vi "Scan_Hopping multiple CV at Surface.vi"() -> ()   [LabVIEW 2023]
uses:
  Sub_Vi/TypeDefs/Settings.ctl
  Sub_Vi/TypeDefs/ChangeOnFly.ctl
  Sub_Vi/TypeDefs/Display.ctl
  Sub_Vi/TypeDefsControls/Feedback Type.ctl
  Sub_Vi/TypeDefsControls/Time.ctl
  Settings.vi
panel:
  in  "No. of Cycles":i32=1 min=0
  in  "Feedback Type":T1
  in  "ABSOLUTE Distance To Retrack \nat line end /um":dbl=1.0
  out "Estimated Time (mins)":dbl
  in  "Retract After Scan":bool=TRUE
  in  "Post CV Time / s":dbl
  in  "Post Clean _Pre CV Time / s":dbl
  in  "Clean Time / s":dbl
  in  "V 4":dbl
  in  "V 3":dbl
  in  "Input Cluster":T2={"Scan Rate (um/s)"=15.0, "X Start"=15.0, "X End"=15.0, "Y Start"=15.0, "Y End"=15.0, " Z Start"=15.0, "HoppingDistance"=1.0, "V"=15.0, "Z End"=15.0, "Approach Rate Hopping (um/s)"=15.0, "Retrack Rate (um/s)"=15.0, "V 2"=15.0, "Approach Rate (um/s)"=15.0, "V 3"=15.0, "CV Rate / V/s"=15.0, "V 4"=15.0, "V 1"=15.0, "HoldTime1/s"=15.0, "Hold time 2 / s"=15.0, "Hold time 3/ s"=15.0, "No. of Cycles"=15}
  in  "Display Cluster":T3
  in  "ChangeonFly":T4
  in  "SettingsCluster":T5={"Sample Rate (us)"=1, "Samples Per Data Point (int, power of 2)"=1000, "DistanceToBulk (um)"=1000.0, "HoldTimeScaler"=0, "SaveData"=TRUE, "DistanceToBulk (um) 2"=-1.0, "DistanceToBulk (um) 3"=-1.0}
  in  "Greater Than":bool=TRUE
  out "XY Graph 3":cluster{"Y":dbl[], "Y":dbl[]}[](graph)
  out "XY Graph 2":cluster{"Y":dbl[], "Y":dbl[]}[](graph)
  in  "CV Rate / V/s":dbl=0.1 min=0.0
  in  "V2":dbl=1.0
  in  "V1":dbl
  in  "Approach Rate Hopping (um/s)":dbl=1.0
  in  "Retrack Rate (um/s)":dbl=1.0
  in  "HoppingDistance":dbl=1.0
  in  "Z End":dbl=38.0
  in  "ABSOLUTE Distance To Retrack / um":dbl=1.0
  in  "Upper dZ limit":i32=8
  in  "Feedback Threshold\nAbsolute value":dbl=1e-13
  in  "P":fxp<+/-,32,1> format="%.32g"
  in  "X Center":dbl=150.0 min=0.0 max=300.0
  in  "Y Center":dbl=150.0 min=0.0 max=300.0
  in  "Y Width":dbl=10.0
  in  "X Width":dbl=10.0
  in  "Scan Rate (um/s)":dbl=1.0
  in  "V":dbl=1.0
  in  "Approach Rate (um/s)":dbl=1.0
  in  "Z Start height":dbl
  in  "Start scan Button":bool
  in  "Stop":bool
  in  "Pause":bool
  in  "Start Scanning Button":bool
  out "Y end":dbl
  out "X end":dbl
  out "X start":dbl
  out "Y start":dbl
  in  "Tab Control 4":T6(tab)
  out "Topography":dbl[][](graph)
  out "Current 1":dbl[][](graph)
  out "Current 2":dbl[][](graph)
  out "Current 3":dbl[][](graph)
  out "Waveform Graph 2":dbl[](graph)
  out "Waveform Graph":dbl[](graph)
  out "XY Graph":cluster{"Y":dbl[], "Y":dbl[]}[](graph)
  out "Waveform Graph 4":dbl[](graph)
  out "Waveform Graph 3":dbl[](graph)
  # "Feedback  Settings"
  # "Approach  Settings"
  # "Scan  Settings"
  # "CV rate must not be zero"
  # "Define Scan area \nAbout centre"
  # "No. of Cycles"
  # "V3"
  # "V1"
  # "Clean Time / s"
  # "V"
  # "V"
  # "Jump to V"
  # "Approach"
  # "CV Rate"
  # "CV Rate"
  # "Post CV Time"
  # "Retract"
  # "V2"
  # "Post Clean Pre CV Time"
  # "V2"
  # "V4"
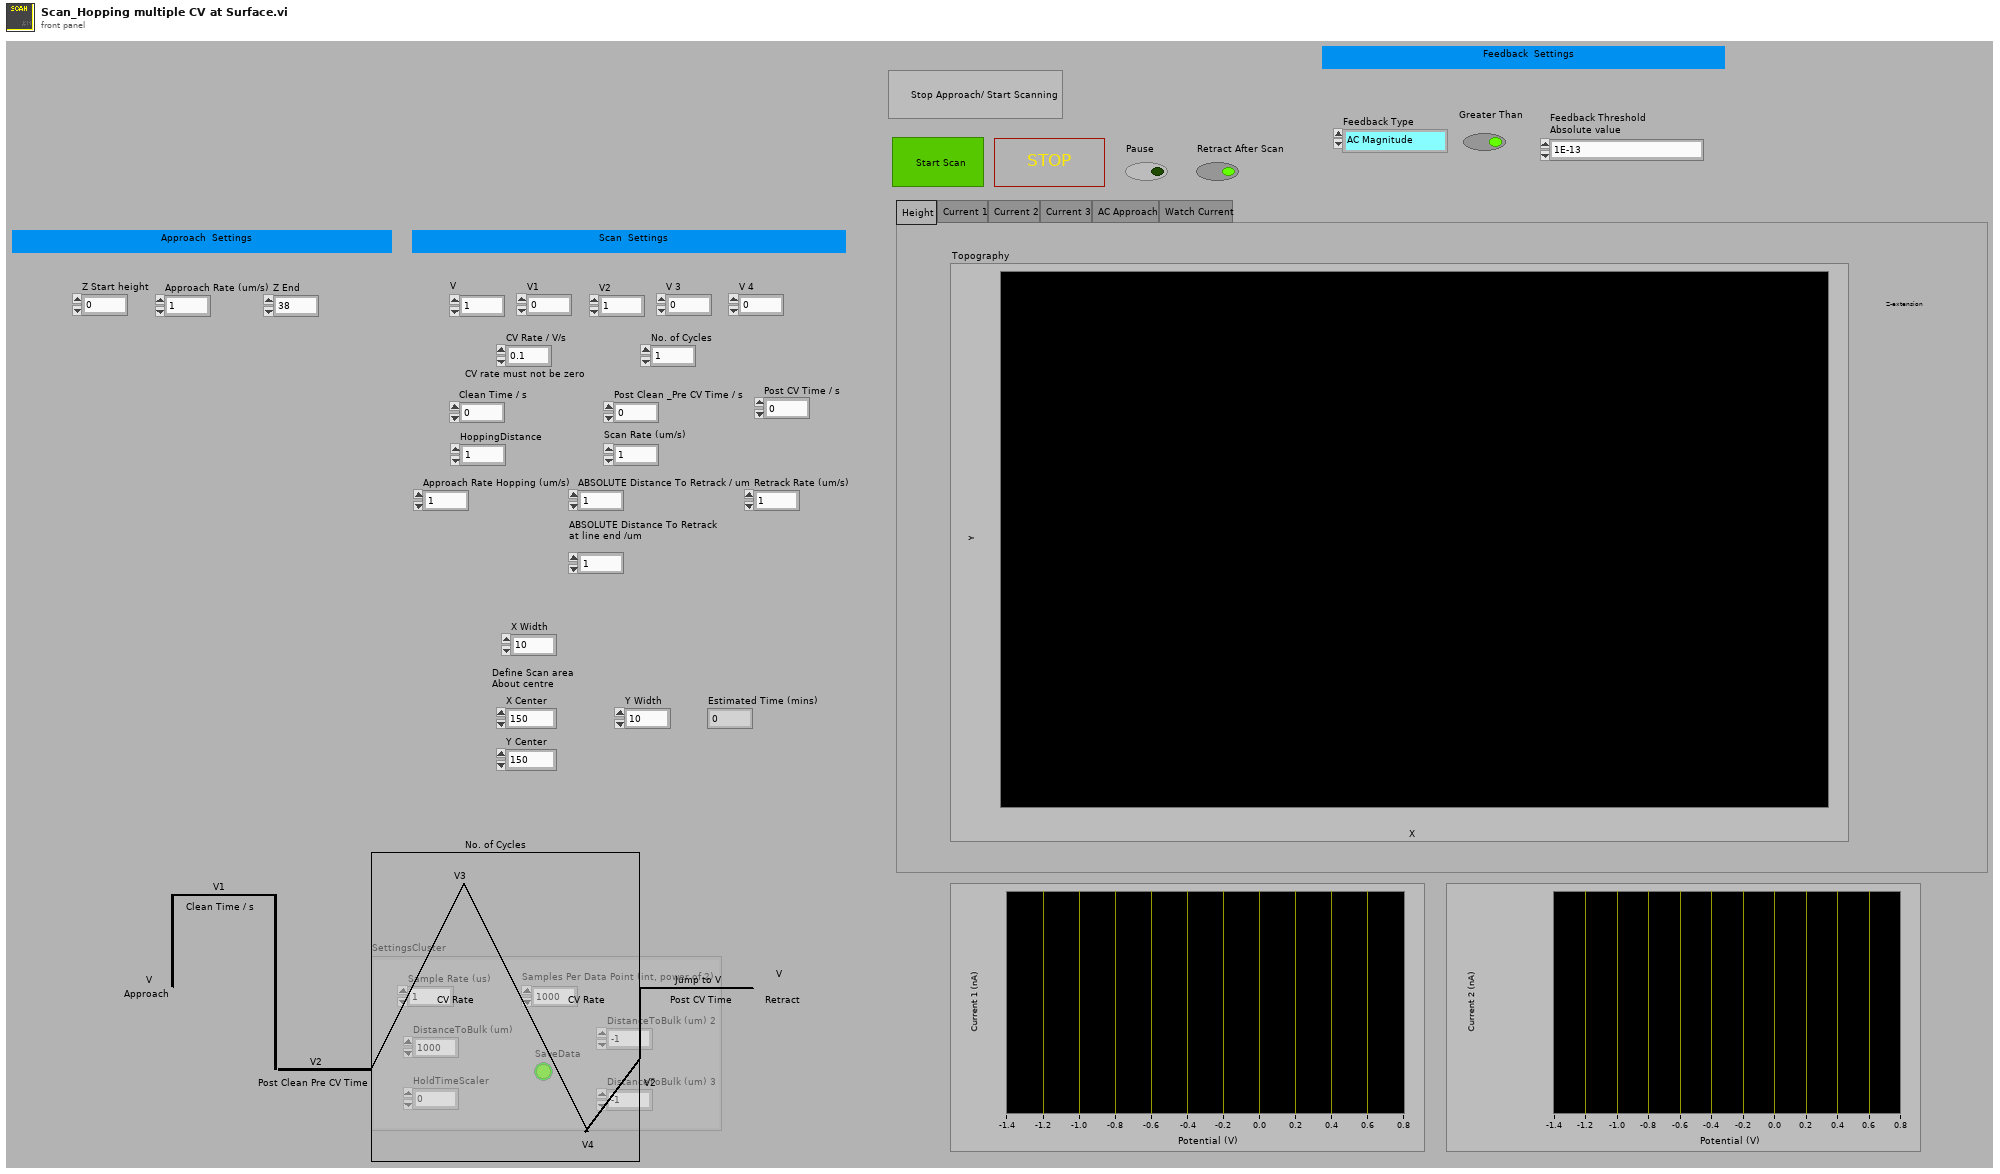
[diagram p1: front panel]
types:
  T1 = typedef "Feedback Type.ctl" = enum16{"AC Magnitude", "Current 1", "Current 2", "Phase"}
  T2 = cluster{"Scan Rate (um/s)":dbl, "X Start":dbl, "X End":dbl, "Y Start":dbl, "Y End":dbl, " Z Start":dbl, "HoppingDistance":dbl, "V":dbl, "Z End":dbl, "Approach Rate Hopping (um/s)":dbl, "Retrack Rate (um/s)":dbl, "V 2":dbl, "Approach Rate (um/s)":dbl, "V 3":dbl, "CV Rate / V/s":dbl, "V 4":dbl, "V 1":dbl, "HoldTime1/s":dbl, "Hold time 2 / s":dbl, "Hold time 3/ s":dbl, "No. of Cycles":i32}
  T3 = typedef "Display.ctl" = cluster{"X":refnum<vi>, "Y":refnum<vi>, "Z":refnum<vi>, "Amp":refnum<vi>, "Phase":refnum<vi>, "t vs Z":refnum<vi>, "t vs C1":refnum<vi>, "t vs C2":refnum<vi>, "t vs C3":refnum<vi>, "t vs Amp":refnum<vi>, "t vs Phase":refnum<vi>, "t vs X":refnum<vi>, "t vs Y":refnum<vi>, "Z vs C1":refnum<vi>, "Z vs C2":refnum<vi>, "Z vs C3":refnum<vi>, "V vs C1":refnum<vi>, "V vs C2":refnum<vi>, "V vs C3":refnum<vi>, "X/Y/Z F":refnum<vi>, "X/Y/Z R":refnum<vi>, "X/Y/C1 F":refnum<vi>, "X/Y/C1 R":refnum<vi>, "X/Y/C2 F":refnum<vi>, "X/Y/C2 R":refnum<vi>, "X/Y/C3 F":refnum<vi>, "X/Y/C3 R":refnum<vi>, "NumberOfLines":u16, "um Per Pixel":dbl, "um Per Line":dbl, "X Center":dbl, "Hop X/Y/Z":refnum<vi>, "Hop X/Y/C1":refnum<vi>, "Hop X/Y/C2":refnum<vi>, "Hop X/Y/C3":refnum<vi>, "X Width":dbl, "Y Width":dbl, "Hopping Distance":dbl, "V2 vs C1":refnum<vi>, "V vs Phase":refnum<vi>, "Y Center":dbl, "Number of Pixels":dbl, "V2 vs C2":refnum<vi>, "V2 vs C3":refnum<vi>, "V vs y":refnum<vi>, "V2 vs y":refnum<vi>, "Z vs Amp":refnum<vi>, "Z vs Phase":refnum<vi>}
  T4 = typedef "ChangeOnFly.ctl" = cluster{"Stop (boolean)":refnum<vi>, "Pause (boolean)":refnum<vi>, "EndCurrentLine (boolean)":refnum<vi>, "max movement per update step (Interger, nm)":refnum<vi>, "P (float, arb)":refnum<vi>, "Feedback set point (double, Amps)":refnum<vi>, "Voltage (double, V)":refnum<vi>, "Feedback set point 2 (double, Amps)":refnum<vi>, "Stop on Greater Than 2? (boolean)":refnum<vi>, "Stop on Greater Than? (boolean)":refnum<vi>, "Voltage 2 (double, V)":refnum<vi>, "Feedback Type (enum)":refnum<vi>, "Feedback Type 2 (enum)":refnum<vi>}
  T5 = typedef "Settings.ctl" = cluster{"Sample Rate (us)":u32, "Samples Per Data Point (int, power of 2)":i16, "DistanceToBulk (um)":dbl, "HoldTimeScaler":u64, "SaveData":bool, "DistanceToBulk (um) 2":dbl, "DistanceToBulk (um) 3":dbl}
  T6 = enum32{"Height", "Current 1", "Current 2", "Current 3", "AC Approach", "Watch Current"}
  T7 = typedef "Time.ctl" = dbl
  T8 = typedef "WayPointCluster.ctl" = cluster{"X (um)":dbl[], "Y (um)":dbl[], "Z (um)":dbl[], "V (V)":dbl[], "X Velocity (um s-1)":dbl[], "Y Velocity (um s-1)":dbl[], "Z Velocity (um s-1)":dbl[], "V Velocity (V s-1)":dbl[], "FeedBack Type (enum)":u16[], "Move X (boolean)":bool[], "Move Y (boolean)":bool[], "Move Z (boolean)":bool[], "Move V (boolean)":bool[], "Jump V (boolean)":bool[], "Hold (boolean)":bool[], "Hold Time":u32[], "V2 (V)":dbl[], "Move V2":bool[], "V2 Velocity (V s-1)":dbl[], "Jump V2 (boolean)":bool[], "Update z Position delta (ms)":i16[], "Hold Feedback1":bool[], "Move Z PicoMotor":bool[], " Z PicoMotor Direction":bool[], "DIO0":bool[]}
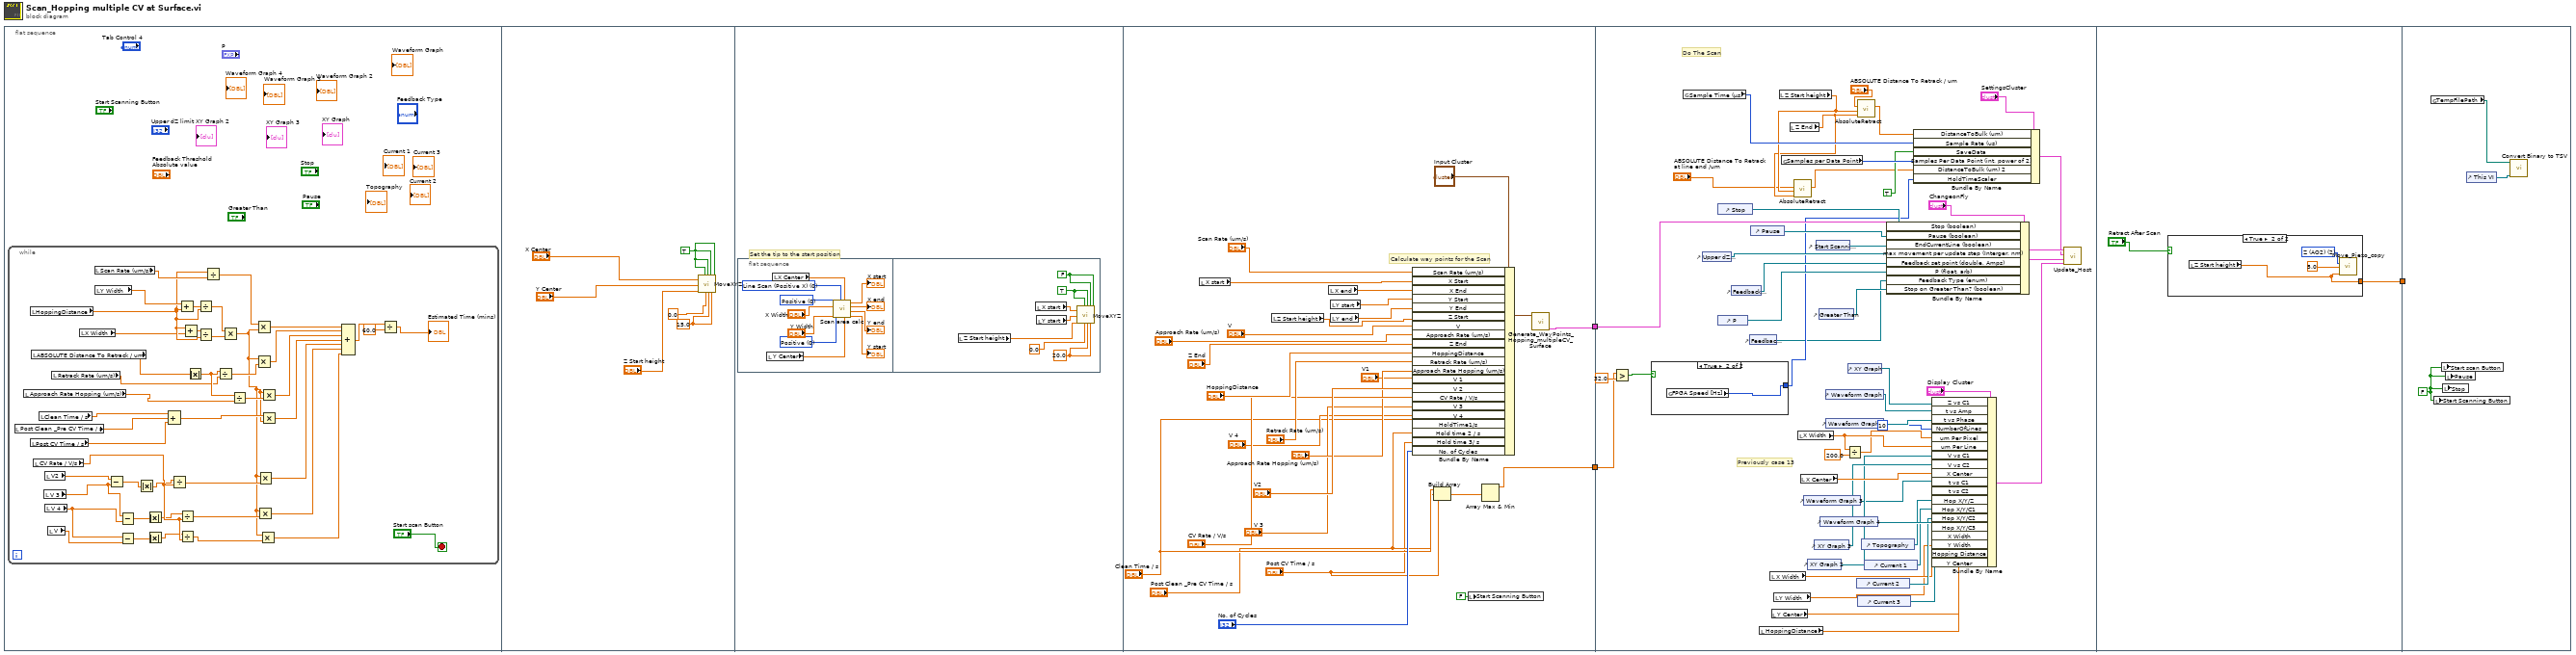
[diagram p0: block diagram]
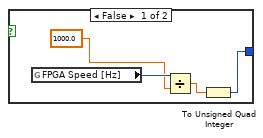
[diagram p2: hidden frame]
diagram:
  n1 = flat-sequence {
    tunnel: [w86] -> w3
    tunnel: [w73] -> w1
    tunnel: w3 -> [w112]
    tunnel: w1 -> [w101]
    tunnel: [w154] -> w2
    tunnel: w2 -> [_]
    frame #0 {
      n2 = while {
        stop <- "Start scan Button" stop-if-true
        n3 = local read "Post Clean _Pre CV Time / s"() -> (w17:dbl)
        n4 = local read "Approach Rate Hopping (um/s)"() -> (w20:dbl)
        n5 = local read "HoppingDistance"() -> (w23:dbl)
        n6 = local read "Post CV Time / s"() -> (w16:dbl)
        n7 = local read "ABSOLUTE Distance To Retrack / um"() -> (w21:dbl)
        n8 = local read "CV Rate / V/s"() -> (w7:dbl)
        n9 = local read "Clean Time / s"() -> (w18:dbl)
        n10 = local read "V 3"() -> (w14:dbl)
        n11 = local read "V2"() -> (w15:dbl)
        n12 = local read "V 4"() -> (w10:dbl)
        n13 = local read "V"() -> (w11:dbl)
        n14 = local read "Retrack Rate (um/s)"() -> (w19:dbl)
        n15 = local read "X Width"() -> (w22:dbl)
        n16 = local read "Scan Rate (um/s)"() -> (w25:dbl)
        n17 = local read "Y Width"() -> (w24:dbl)
        n18 = Subtract(x=w15, y=w14) -> (x-y=w42:dbl)
        n19 = Subtract(x=w14, y=w10) -> (x-y=w41:dbl)
        n20 = Subtract(x=w10, y=w11) -> (x-y=w13:dbl)
        n21 = Absolute Value(x=w42) -> (abs(x)=w4:dbl)
        n22 = Absolute Value(x=w41) -> (abs(x)=w5:dbl)
        n23 = Absolute Value(x=w13) -> (abs(x)=w6:dbl)
        n24 = Compound Arithmetic op=ADD(w18, w17, w16) -> (w40:dbl)
        n25 = Divide(x=w4, y=w7) -> (x/y=w43:dbl)
        n26 = Add(x=w24, y=w23) -> (x+y=w29:dbl)
        n27 = Divide(x=w5, y=w7) -> (x/y=w44:dbl)
        n28 = Divide(x=w6, y=w7) -> (x/y=w9:dbl)
        n29 = Add(x=w23, y=w22) -> (x+y=w28:dbl)
        n30 = Absolute Value(x=w21) -> (abs(x)=w30:dbl)
        n31 = Divide(x=w29, y=w23) -> (x/y=w27:dbl)
        n32 = Divide(x=w28, y=w23) -> (x/y=w26:dbl)
        n33 = Divide(x=w23, y=w25) -> (x/y=w33:dbl)
        n34 = Divide(x=w30, y=w19) -> (x/y=w35:dbl)
        n35 = Multiply(x=w27, y=w26) -> (x*y=w12:dbl)
        n36 = Divide(x=w30, y=w20) -> (x/y=w31:dbl)
        n37 = Multiply(x=w33, y=w12) -> (x*y=w34:dbl)
        n38 = Multiply(x=w12, y=w35) -> (x*y=w36:dbl)
        n39 = Multiply(x=w12, y=w44) -> (x*y=w47:dbl)
        n40 = Multiply(x=w12, y=w43) -> (x*y=w46:dbl)
        n41 = Multiply(x=w12, y=w9) -> (x*y=w8:dbl)
        n42 = Multiply(x=w12, y=w31) -> (x*y=w32:dbl)
        n43 = Multiply(x=w40, y=w12) -> (x*y=w45:dbl)
        n44 = Compound Arithmetic op=ADD(w34, w36, w32, w45, w46, w47, w8) -> (w37:dbl)
        n45 = Divide(x=w37, y=60.0) -> (x/y=→"Estimated Time (mins)":dbl)
      }
    }
    frame #1 {
      w53 = TRUE ("Set X")
      w54 = 15.0 ("Scan Rate (V/s) X and Y")
      n46 = call "MoveXYZ.vi"("X final height"="X Center", "Y final height"="Y Center", "Z final height"="Z Start height", "Set X"=w53, "V final"=0.0 ("Z initial height"), "Set Y"=w53, "Scan Rate (um/s)"=w54, "Set Z"=w53, "Scan Rate (V/s) 2"=w54, "Set Voltage"=w53) -> ()  [unwired: 10 in]
    }
    frame #2 {
      # "Set the tip to the start position"
      n47 = flat-sequence {
        frame #0 {
          w55 = u16 0 items=["Positive", "Negative"] ("Major Axis Direction")
          w56 = u16 0 items=["Positive", "Negative"] ("Minor Axis Direction")
          w57 = u16 0 items=["Line Scan (Positive X)", "Line Scan (Negative X)", "Line Scan (Positive Y)", "Line Scan (Negative Y)"] ("Scan Type")
          n48 = local read "Y Center"() -> (w58:dbl)
          n49 = local read "X Center"() -> (w59:dbl)
          n50 = call "Scan area calc.vi"("Y Width"="Y Width", "Major Axis Direction"=w55, "X Width"="X Width", "Minor Axis Direction"=w56, "Scan Type"=w57, "Y Center"=w58, "X Center"=w59) -> ("Y start"=→"Y start":dbl, "Y end"=→"Y end":dbl, "X end"=→"X end":dbl, "X start"=→"X start":dbl)
        }
        frame #1 {
          w68 = FALSE ("Set Z")
          w69 = TRUE ("Set X")
          w70 = 20.0 ("Scan Rate (V/s)")
          n51 = local read "Z Start height"() -> (w66:dbl)
          n52 = local read "X start"() -> (w72:dbl)
          n53 = local read "Y start"() -> (w71:dbl)
          n54 = call "MoveXYZ.vi"("X final height"=w72, "Y final height"=w71, "Z final height"=w66, "Set X"=w69, "V final"=0.0 ("Scan Rate (V/s) X and Y"), "Set Y"=w69, "Scan Rate (um/s)"=w70, "Set Z"=w68, "Scan Rate (V/s) 2"=w70, "Set Voltage"=w68) -> ()  [unwired: 10 in]
        }
      }
    }
    frame #3 {
      # "Calculate way points for the Scan"
      n55 = local read "X start"() -> (w98:dbl)
      n56 = local read "Z Start height"() -> (w91:dbl)
      n57 = local read "X end"() -> (w97:dbl)
      n58 = local read "Y start"() -> (w99:dbl)
      n59 = local read "Y end"() -> (w96:dbl)
      n60 = Bundle By Name(cluster="Input Cluster", "Scan Rate (um/s)"="Scan Rate (um/s)", "X Start"=w98, "X End"=w97, "Y Start"=w99, "Y End"=w96, "Z Start"=w91, "V"="V", "Approach Rate (um/s)"="Approach Rate (um/s)", "Z End"="Z End", "HoppingDistance"="HoppingDistance", "Retrack Rate (um/s)"="Retrack Rate (um/s)", "Approach Rate Hopping (um/s)"="Approach Rate Hopping (um/s)", "V 1"="V1", "V 2"="V2", "CV Rate / V/s"="CV Rate / V/s", "V 3"="V 3", "V 4"="V 4", "HoldTime1/s"="Clean Time / s", "Hold time 2 / s"="Post Clean _Pre CV Time / s", "Hold time 3/ s"="Post CV Time / s", "No. of Cycles"="No. of Cycles") -> (w83:T2)
      n61 = Build Array("Clean Time / s", "Post Clean _Pre CV Time / s", "Post CV Time / s") -> (w74:dbl[])
      n62 = local write "Start Scanning Button"(FALSE ("Start Scanning Button")) -> ()
      n63 = Array Max & Min(array=w74) -> (max value=w73:dbl)  [unwired: 3 out]
      n64 = call "Generate_WayPoints_Hopping_multipleCV_Surface.vi"("Input Cluster"=w83) -> ("output cluster"=w86:T8)  [unwired: 10 in]
    }
    frame #4 {
      # "Previously case 13"
      # "Do The Scan"
      n65 = Greater?(x=w101, y=T7 32.0) -> (0:w103:bool)
      n66 = case shown="True" w103 {
        tunnel: [w148 w152] -> w102
        frame False {
          n67 = global read "Settings.vi" "FPGA Speed [Hz]"() -> (w151:i64)
          n68 = Divide(x=w151, y=1000.0) -> (x/y=w149:dbl)
          n69 = To Unsigned Quad Integer(1:w149) -> (0:w148:u64)
        }
        frame True {
          n70 = global read "Settings.vi" "FPGA Speed [Hz]"() -> (w152:i64)
        }
      }
      n71 = global read "Settings.vi" "Sample Time (µs)"() -> (w113:u32)
      n72 = control-ref of="Upper dZ limit"() -> (w141:refnum<vi>)
      n73 = control-ref of="P"() -> (w140:refnum<vi>)
      n74 = control-ref of="Stop"() -> (w137:refnum<vi>)
      n75 = control-ref of="Feedback Threshold\nAbsolute value"() -> (w139:refnum<vi>)
      n76 = control-ref of="Feedback Type"() -> (w100:refnum<vi>)
      n77 = control-ref of="Pause"() -> (w138:refnum<vi>)
      n78 = local read "HoppingDistance"() -> (w115:dbl)
      n79 = local read "X Width"() -> (w117:dbl)
      n80 = local read "Y Center"() -> (w114:dbl)
      n81 = local read "Y Width"() -> (w116:dbl)
      n82 = local read "Z Start height"() -> (w108:dbl)
      n83 = global read "Settings.vi" "Samples per Data Point"() -> (w124:u16)
      n84 = local read "Z End"() -> (w107:dbl)
      n85 = call "AbsoluteRetract.vi"("Z End"=w107, "Z Start height"=w108, "Distance To Retract / um"="ABSOLUTE Distance To Retrack \nat line end /um") -> ("Distance To Retract / um 2"=w105:dbl)  [unwired: 8 in]
      n86 = local read "X Width"() -> (w136:dbl)
      n87 = local read "X Center"() -> (w133:dbl)
      n88 = control-ref of="Waveform Graph 3"() -> (w129:refnum<vi>)
      n89 = control-ref of="XY Graph 2"() -> (w130:refnum<vi>)
      n90 = control-ref of="XY Graph 3"() -> (w131:refnum<vi>)
      n91 = control-ref of="Start Scanning Button"() -> (w142:refnum<vi>)
      n92 = control-ref of="Greater Than"() -> (w123:refnum<vi>)
      n93 = control-ref of="Waveform Graph 4"() -> (w128:refnum<vi>)
      n94 = control-ref of="Waveform Graph"() -> (w146:refnum<vi>)
      n95 = control-ref of="Waveform Graph 2"() -> (w145:refnum<vi>)
      n96 = Divide(x=w136, y=200.0) -> (x/y=w134:dbl)
      n97 = control-ref of="XY Graph"() -> (w147:refnum<vi>)
      n98 = control-ref of="Current 2"() -> (w119:refnum<vi>)
      n99 = control-ref of="Current 3"() -> (w118:refnum<vi>)
      n100 = call "AbsoluteRetract.vi"("Z End"=w107, "Z Start height"=w108, "Distance To Retract / um"="ABSOLUTE Distance To Retrack / um") -> ("Distance To Retract / um 2"=w109:dbl)  [unwired: 8 in]
      n101 = control-ref of="Topography"() -> (w121:refnum<vi>)
      n102 = control-ref of="Current 1"() -> (w120:refnum<vi>)
      n103 = Bundle By Name(cluster="ChangeonFly", "Stop (boolean)"=w137, "Pause (boolean)"=w138, "EndCurrentLine (boolean)"=w142, "max movement per update step (Interger, nm)"=w141, "Feedback set point (double, Amps)"=w139, "P (float, arb)"=w140, "Feedback Type (enum)"=w100, "Stop on Greater Than? (boolean)"=w123) -> (w143:T4)
      n104 = Bundle By Name(cluster="SettingsCluster", "DistanceToBulk (um)"=w109, "Sample Rate (us)"=w113, "SaveData"=TRUE ("Save Data"), "Samples Per Data Point (int, power of 2)"=w124, "DistanceToBulk (um) 2"=w105, "HoldTimeScaler"=w102) -> (w111:T5)
      n105 = Bundle By Name(cluster="Display Cluster", "Z vs C1"=w147, "t vs Amp"=w146, "t vs Phase"=w145, "NumberOfLines"=u16 10, "um Per Pixel"=w134, "um Per Line"=w136, "V vs C1"=w130, "V vs C2"=w131, "X Center"=w133, "t vs C1"=w129, "t vs C2"=w128, "Hop X/Y/Z"=w121, "Hop X/Y/C1"=w120, "Hop X/Y/C2"=w119, "Hop X/Y/C3"=w118, "X Width"=w117, "Y Width"=w116, "Hopping Distance"=w115, "Y Center"=w114) -> (w144:T3)
      n106 = call "Update_Host.vi"("Display Cluster"=w144, "ChangeonFly"=w143, "SettingsCluster"=w111, "WayPointCluster"=w112) -> ()  [unwired: 6 in]
    }
    frame #5 {
      n107 = case shown="True" "Retract After Scan" {
        tunnel: [_ w155] -> w154
        frame False {
        }
        frame True {
          w157 = u16 2 items=["X (AO0)", "Y (AO1)", "Z (AO2)", "V (AO3)"] ("Channel")
          n108 = local read "Z Start height"() -> (w155:dbl)
          n109 = call "Move_Piezo_copy.vi"("Piezo"=w157, "Movement Speed (µm/s)"=5.0 ("Scan Rate (um/s)"), "Position (µm) (or V)"=w155) -> ()  [unwired: 13 in]
        }
      }
    }
    frame #6 {
      w160 = FALSE ("Stop")
      n110 = global read "Settings.vi" "TempFilePath"() -> (w158:path)
      n111 = local write "Start Scanning Button"(w160) -> ()
      n112 = local write "Start scan Button"(w160) -> ()
      n113 = local write "Stop"(w160) -> ()
      n114 = local write "Pause"(w160) -> ()
      n115 = control-ref of="This VI"() -> (w159:refnum<vi>)
      n116 = call "Convert Binary to TSV.vi"("This VI"=w159, "TDMS DataFile Name"=w158) -> ()  [unwired: 10 in]
    }
  }
